vi "gauss-seidel(SubVI).vi"(4 "Tolerancja":dbl, 8 "Initial Guess":dbl[](array[numeric]), 10 "Wektor b":dbl[](array[numeric]), 11 "Macierz A":dbl[][](array[numeric])) -> (2 "Wykonana iczba Iteracji":i32, 3 "Metoda Gaussa-Seidla":dbl[](array[numeric]))   [LabVIEW 2020]
uses:
  <vilib>/Analysis/Matrix/Numeric/Conversions/Array To Matrix - RA2.vi
  <vilib>/Analysis/Matrix/Numeric/Conversions/Array To Matrix - RA.vi
  <vilib>/addons/Multicore Analysis and Sparse Matrix/Linear Algebra/_linalg/Inverse Matrix (DBL).vi
  <vilib>/addons/Multicore Analysis and Sparse Matrix/BLAS/_blas/dgemm - General Matrix-Matrix Product (DBL).vi
  <vilib>/Analysis/Matrix/Numeric/Multiply/Multiply - RM,R.vi
  <vilib>/Analysis/BLAS.llb/dgemv - General Matrix-Vector Product (DBL).vi
  <vilib>/addons/Multicore Analysis and Sparse Matrix/BLAS/_blas/dgemv - General Matrix-Vector Product (DBL).vi
  <vilib>/Analysis/NI_AALBLAS.lvlib
  <vilib>/Analysis/Matrix/NI_Matrix.lvlib
  <vilib>/addons/Multicore Analysis and Sparse Matrix/BLAS/NI_MASM_BLAS.lvlib
  <vilib>/addons/Multicore Analysis and Sparse Matrix/Linear Algebra/NI_MASM_BasicLinAlg.lvlib
panel:
  out "Stop":bool
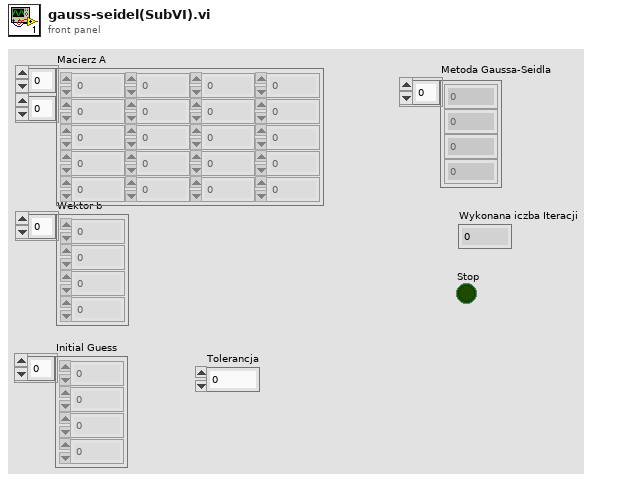
[diagram p1: front panel]
types:
  T1 = typedef "NI_Matrix.lvlib/RealMatrix.ctl" = dbl[][]
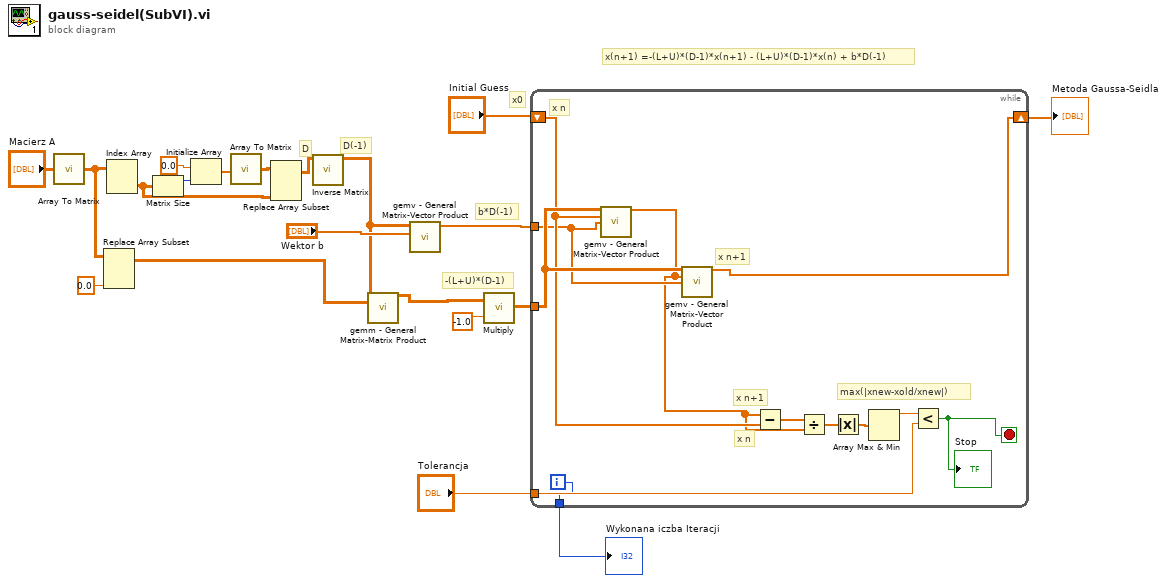
[diagram p0: block diagram]
diagram:
  # "x(n+1) =-(L+U)*(D-1)*x(n+1) - (L+U)*(D-1)*x(n) + b*D(-1)"
  # "b*D(-1)"
  # "-(L+U)*(D-1)"
  # "x0"
  # "D(-1)"
  # "D"
  n1 = call-poly <vilib>:"Array To Matrix.vi"("Real 2D Array"="Macierz A") -> ("Real Matrix"=w13:T1)
  n2 = Replace Array Subset(array=w13, new element=0.0 ("new diagonal/fill element")) -> (w6:T1)  [unwired: 2 in]
  n3 = Index Array(array=w13) -> (element=w7:T1)  [unwired: 2 in]
  n4 = Matrix Size(0:w7) -> (1:w11:i32)  [unwired: 1 out]
  n5 = Initialize Array(0.0 ("element"), w11) -> (w9:dbl[])
  n6 = call-poly <vilib>:"Array To Matrix.vi"("Real 1D Array"=w9) -> ("Real Matrix (Column Vector)"=w8:T1)
  n7 = Replace Array Subset(array=w8, new element=w7) -> (w3:T1)  [unwired: 2 in]
  n8 = call-poly <vilib>:"Inverse Matrix.vi"("Input Matrix"=w3) -> ("Inverse Matrix"=w19:T1)  [unwired: 9 in, 1 out]
  n9 = call-poly <vilib>:"gemm - General Matrix-Matrix Product.vi"("A"=w19, "B"=w6) -> ("dgemm"=w17:T1)  [unwired: 12 in, 1 out]
  n10 = call-poly <vilib>:"gemv - General Matrix-Vector Product.vi"("x"="Wektor b", "A"=w19) -> ("dgemv"=w16:dbl[])  [unwired: 8 in, 1 out]
  n11 = call-poly <vilib>:"Multiply.vi"("Real Scalar c"=-1.0 ("y"), "Real Matrix A"=w17) -> ("A * c"=w5:T1)
  n12 = while {
    tunnel: w16 -> [w23]
    shift-right: [w22] -> w1
    shift-left: "Initial Guess" -> [w24]
    tunnel: [w26] -> w14
    tunnel: w5 -> [w25]
    tunnel: "Tolerancja" -> [w27]
    i -> [w26]
    stop <- w28 stop-if-true
    # "x n+1"
    # "x n"
    # "x n+1"
    # "max(|xnew-xold/xnew|)"
    # "x n"
    n13 = call-poly <vilib>:"gemv - General Matrix-Vector Product.vi"("A"=w25, "x"=w24, "y"=w23) -> ("dgemv"=w21:dbl[])  [unwired: 11 in, 1 out]
    n14 = call-poly <vilib>:"gemv - General Matrix-Vector Product.vi"("A"=w25, "x"=w21, "y"=w23) -> ("dgemv"=w22:dbl[])  [unwired: 11 in, 1 out]
    n15 = Subtract(x=w21, y=w24) -> (x-y=w32:dbl[])
    n16 = Divide(x=w32, y=w21) -> (x/y=w31:dbl[])
    n17 = Absolute Value(x=w31) -> (abs(x)=w30:dbl[])
    n18 = Array Max & Min(array=w30) -> (max value=w29:dbl)  [unwired: 3 out]
    n19 = Less?(x=w29, y=w27) -> (x < y?=w28:bool)
    "Stop" <- w28
  }
  "Metoda Gaussa-Seidla" <- w1
  "Wykonana iczba Iteracji" <- w14
